vi "Save Analysis Result Histogram Color Grade.vi"(8 "error in (no error)":errorcluster, 9 "Include Histogram Statistics (F: Disable)":bool, 10 "Include Color Grade Data (F: Disable)":bool, 11 "VISA resource name":refnum<visa-resource-name>) -> (0 "error out":errorcluster, 3 "VISA resource name out":refnum<visa-resource-name>)   [LabVIEW 2016, in "Agilent 2000 3000 X-Series.lvlib"]
doc: "Enables or Disables including color grade and histogram data in the saved file. Call <b>Save Analysis Result</b> after this VI to save to a file.\n\n<b>Note:</b>\nThis VI is specific to the 6000-X Series oscilloscopes. These features are not available on other models."
uses:
  Agilent 2000 3000 X-Series.lvlib
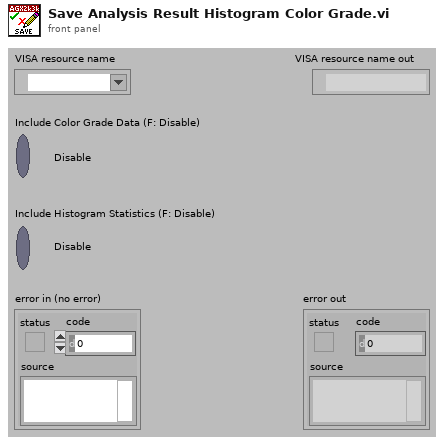
[diagram p1: front panel]
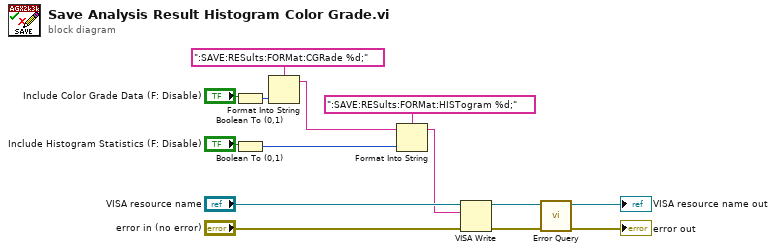
[diagram p0: block diagram]
diagram:
  n1 = Boolean To (0,1)(Boolean="Include Color Grade Data (F: Disable)") -> (0, 1=w12:i16)
  n2 = Boolean To (0,1)(Boolean="Include Histogram Statistics (F: Disable)") -> (0, 1=w10:i16)
  n3 = Format Into String(format string=":SAVE:RESults:FORMat:CGRade %d;", w12) -> (resulting string=w1:string)  [unwired: 2 in, 1 out]
  n4 = Format Into String(format string=":SAVE:RESults:FORMat:HISTogram %d;", initial string=w1, w10) -> (resulting string=w6:string)  [unwired: 1 in, 1 out]
  n5 = VISA Write(VISA resource name="VISA resource name", write buffer=w6, error in (no error)="error in (no error)") -> (VISA resource name out=w5:refnum<visa-resource-name>, error out=w4:errorcluster)  [unwired: 1 out]
  n6 = call "Error Query.vi"("error in (no error)"=w4, "VISA resource name"=w5) -> ("error out"=→"error out":errorcluster, "VISA resource name out"=→"VISA resource name out":refnum<visa-resource-name>)  [unwired: 6 in, 2 out]
